vi "Get points for single shot.vi"(7 "error in (no error)":errorcluster) -> (0 "error out":errorcluster, 2 "Number of Points 2":dbl)   [LabVIEW 2015, in "Gage digitizer actor.lvclass"]
uses:
  Gage digitizer actor.lvclass
panel:
  in  "Number of Points":dbl=8640.0 min=160.0 step=160.0
  in  "Press when finished":bool=TRUE
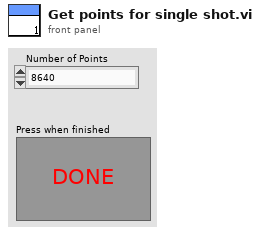
[diagram p1: front panel]
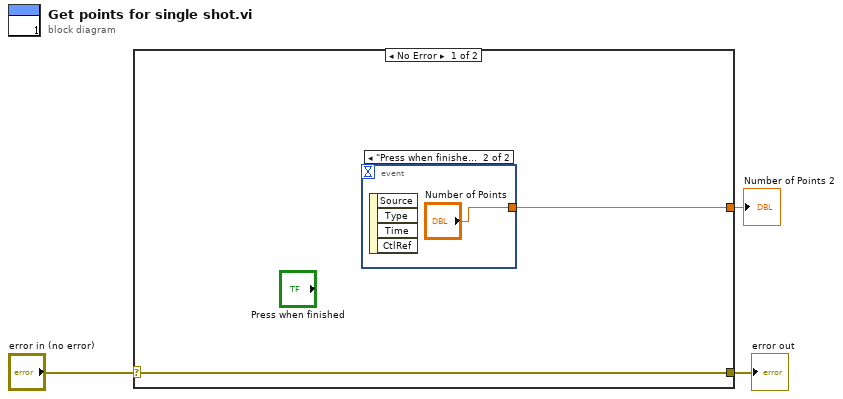
[diagram p0: block diagram]
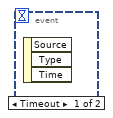
[diagram p2: hidden frame]
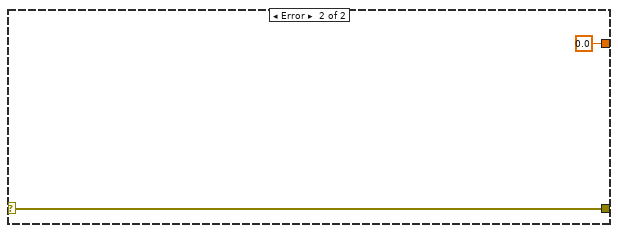
[diagram p3: hidden frame]
diagram:
  n1 = case shown="No Error" "error in (no error)" {
    selector: "error in (no error)" -> [w5 w8]
    tunnel: [w5 w8] -> w2
    tunnel: [w4 0.0 ("Number of Points")] -> w1
    frame No Error {
      n2 = event shown="[1] \"Press when finished\": Value Change" {
        selector: _ -> [_ _]
        dyn-events: _ -> [_ _]
        timeout: _ -> [_ _]
        tunnel: [_ "Number of Points"] -> w4
        event Timeout {
          n3 = event-data() -> ()  [unwired: 1 in, 3 out]
        }
        event "Press when finished": Value Change {
          n4 = event-data() -> ()  [unwired: 1 in, 4 out]
        }
      }
    }
    frame Error {
    }
  }
  "error out" <- w2
  "Number of Points 2" <- w1
